vi "SISTEMA INTELIGENTE DE DETECÇÃO DE GAS.vi"() -> ()   [LabVIEW 2020]
uses:
  <vilib>/MakerHub/LINX/Public/Peripherals/Analog/Analog Read 1 Chan.vi
  <vilib>/MakerHub/LINX/Public/Peripherals/Digital/Digital Write 1 Chan.vi
  <vilib>/MakerHub/LINX/Public/Peripherals/Analog/Analog Read N Chans.vi
  <vilib>/MakerHub/LINX/Public/Peripherals/Digital/Digital Write N Chans.vi
  <vilib>/MakerHub/LINX/Private/Local IO/LinxAnalogRead.vi
  <vilib>/MakerHub/LINX/Public/Utilities/Check Channel.vi
  <vilib>/MakerHub/LINX/Private/Local IO/LinxDigitalWrite.vi
  <vilib>/MakerHub/LINX/Public/Utilities/Open Serial.vi
  <vilib>/MakerHub/LINX/Private/Utilties/Generate Error.vi
  <vilib>/MakerHub/LINX/Public/Sensors/Temperature/TMP3x/TMP35.vi
  <vilib>/MakerHub/LINX/LMH-LINX.lvlib
  <vilib>/MakerHub/LINX/Public/Sensors/Temperature/TMP3x/TMP3x.lvlib
panel:
  in  "Tab Control":enum32{"Supervisório", "Configuração"}(tab)
  out "Gráfico da temperatura ambiente":dbl(graph)
  out "2D Picture":picture
  out "Gráfico de gás no ambiente":T1(graph)
  out "ledExp2":bool
  out "ledDep2":bool
  out "ledCoz2":bool
  out "ledCoz1":bool
  out "ledExp1":bool
  out "ledDep1":bool
  out "°C":dbl format="%#_2g"
  out "Cozimento":dbl(knob) scale=0.0..5.0
  out "Expedição":dbl(knob) scale=0.0..5.0
  out "Depósito":dbl(knob) scale=0.0..5.0
  out "Temperatura\nambiente":dbl(slide) scale=0.0..100.0
  out "'ppm'":dbl format="%#_2g"
  out "'ppm'":dbl format="%#_2g"
  out "'ppm'":dbl format="%#_2g"
  in  "fundoAlarme":string
  in  "Set-point gas":fxp<+,64,32>
  in  "Serial Port":refnum<visa-resource-name>="N/A"
  in  "sensorGas1":u8
  in  "sensorGas2":u8
  in  "sensorGas3":u8
  in  "sensorTempLM35":u8
  in  "stop":bool
  in  "saidaSirene":u8
  in  "saidaLuminoso":u8
  in  "diretorioDatalogger":path
  in  "imagemAlertaTemp":path
  in  "Set-point temp":dbl
  in  "imagemNormalidade":path
  in  "imagemAlertaGasTemp":path
  in  "imagemAlertaGas":path
  # "SISTEMA DE MONITORAMENTO DE EMERGÊNCIA"
  # "Planta baixa fábrica alimentícia"
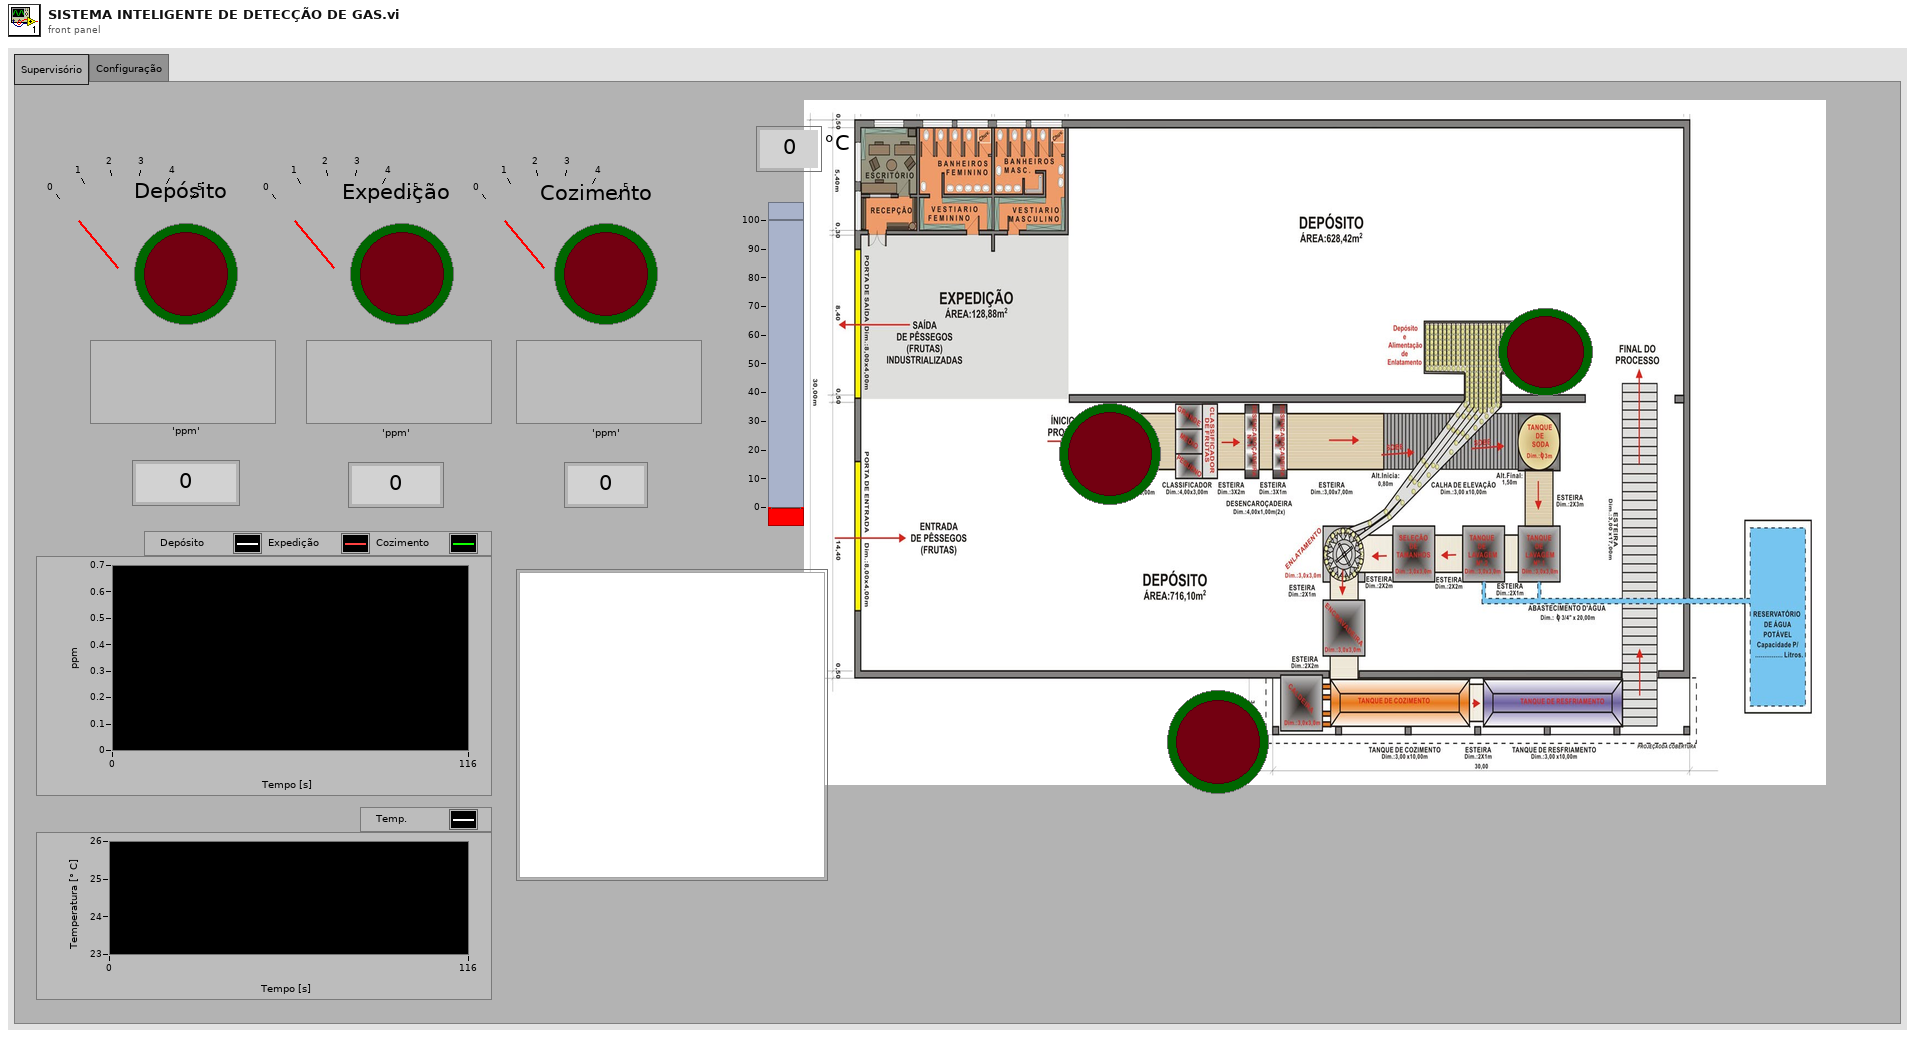
[diagram p1: front panel]
types:
  T1 = cluster{"Depósito":dbl, "Expedição":dbl, "Cozimento":dbl}
  T2 = typedef "LMH-LINX.lvlib/LINX Ref.ctl" = cluster{"IO":T3, "Interface":T4, "LINX Device Config":T5}
  T3 = typedef "LMH-LINX.lvlib/Platform.ctl" = enum16{"Remote", "Local"}
  T4 = typedef "LMH-LINX.lvlib/Interface.ctl" = enum16{"Serial", "TCP"}
  T5 = typedef "LMH-LINX.lvlib/Device.lvlib/LINX Device Config.ctl" = cluster{"Interface":T4, "COM Port":refnum<visa-resource-name>, "TCP Configuration":T6, "Device Family":u8, "Device ID":u8, "Device Name":string, "TCP Ref":refnum<k5>, "Channels":T7}
  T6 = typedef "LMH-LINX.lvlib/Device.lvlib/TCP Config.ctl" = cluster{"IP Address":string, "Port":u16}
  T7 = typedef "LMH-LINX.lvlib/Channels.ctl" = cluster{"DI":u8[], "DO":u8[], "AI":u8[], "AO":u8[], "PWM":u8[], "QE":u8[], "UART":u8[], "I2C 2":u8[], "SPI":u8[], "CAN":u8[], "Servo":u8[], "AI Ref (V)":dbl, "AI Resolution (Bits)":u8, "AO Ref (V)":dbl, "AO Resolution (Bits)":u8}
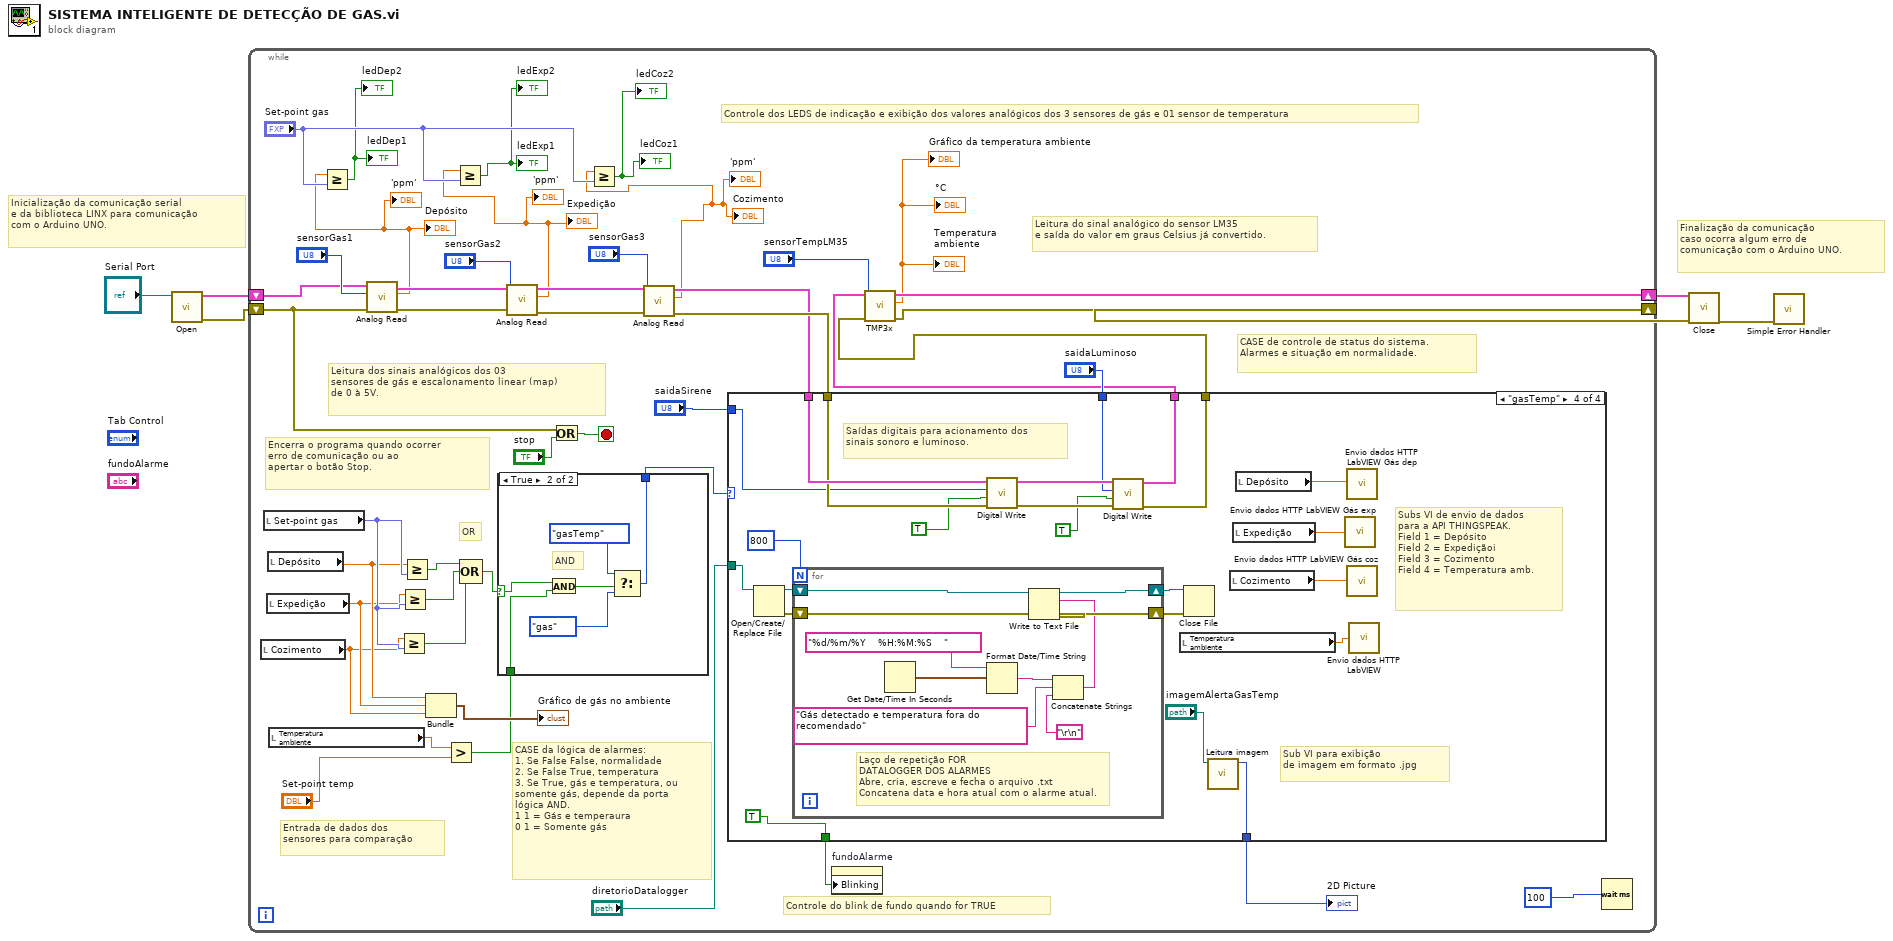
[diagram p0: block diagram]
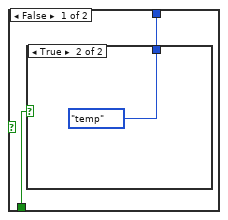
[diagram p2: hidden frame]
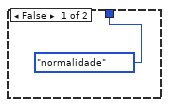
[diagram p3: hidden frame]
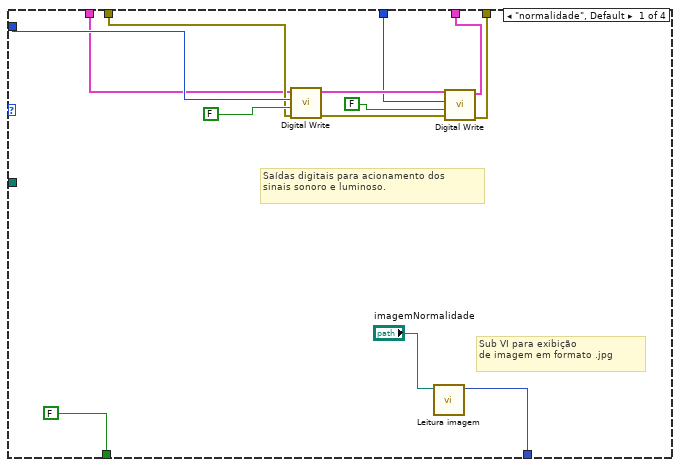
[diagram p4: hidden frame]
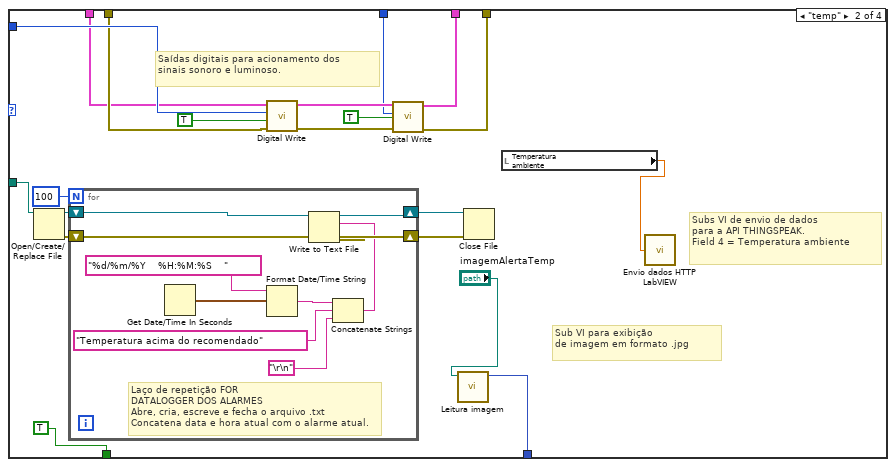
[diagram p5: hidden frame]
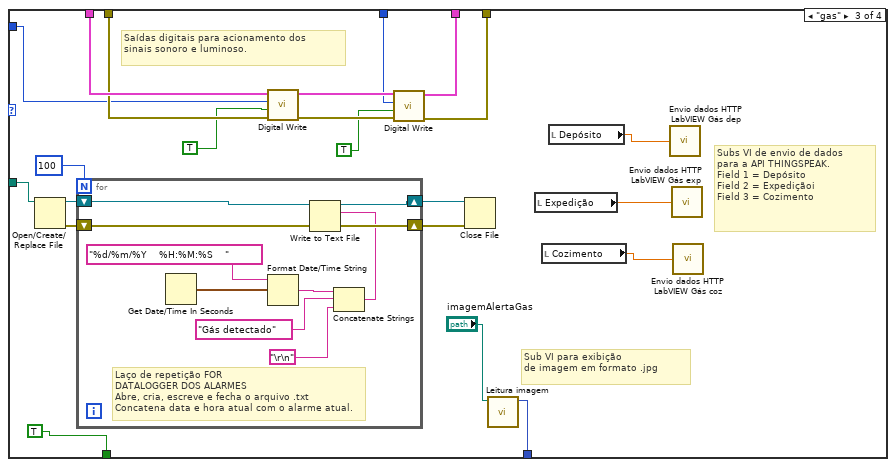
[diagram p6: hidden frame]
diagram:
  # "Finalização da comunicação\ncaso ocorra algum erro de\ncomunicação com o Arduino UNO."
  # "Inicialização da comunicação serial\ne da biblioteca LINX para comunicação \ncom o Arduino UNO."
  n1 = call-poly <vilib>:"Open.vi"("Serial Port"="Serial Port") -> ("Error Out"=w6:errorcluster, "LINX Resource"=w3:T2)  [unwired: 8 in, 1 out]
  n2 = while {
    shift-right: [w50] -> w5
    shift-left: w6 -> [w33]
    shift-right: [w49] -> w2
    shift-left: w3 -> [w34]
    stop <- w48 stop-if-true
    # "Encerra o programa quando ocorrer \nerro de comunicação ou ao \napertar o botão Stop."
    # "Entrada de dados dos\nsensores para comparação"
    # "OR"
    # "CASE de controle de status do sistema. \nAlarmes e situação em normalidade."
    # "Leitura do sinal analógico do sensor LM35 \ne saída do valor em graus Celsius já convertido."
    # "Leitura dos sinais analógicos dos 03\nsensores de gás e escalonamento linear (map)\nde 0 à 5V."
    # "CASE da lógica de alarmes:\n1. Se False False, normalidade\n2. Se False True, temperatura\n3. Se True, gás e temperatura, ou\nsomente gás, depende da porta\nlógica AND.\n1 1 = Gás e temperaura\n0 1 = Somente gás"
    # "Controle do blink de fundo quando for TRUE"
    # "Controle dos LEDS de indicação e exibição dos valores analógicos dos 3 sensores de gás e 01 sensor de temperatura"
    n3 = local read "Cozimento"() -> (w27:dbl)
    n4 = local read "Set-point gas"() -> (w30:fxp<+,64,32>)
    n5 = local read "Expedição"() -> (w28:dbl)
    n6 = local read "Depósito"() -> (w29:dbl)
    n7 = local read "Temperatura\nambiente"() -> (w23:dbl)
    n8 = call-poly <vilib>:"Analog Read.vi"("Error In"=w33, "Analog Channel"="sensorGas1", "LINX Resource"=w34) -> ("Error Out"=w51:errorcluster, "Voltage"=w9:dbl, "LINX Resource"=w45:T2)  [unwired: 5 in, 1 out]
    "Depósito" <- w9
    "'ppm'" <- w9
    n9 = Greater Or Equal?(x=w9, y="Set-point gas") -> (x >= y?=→"ledDep1" →"ledDep2":bool)
    n10 = Greater Or Equal?(x=w27, y=w30) -> (x >= y?=w14:bool)
    n11 = Greater Or Equal?(x=w28, y=w30) -> (x >= y?=w15:bool)
    n12 = Greater Or Equal?(x=w29, y=w30) -> (x >= y?=w16:bool)
    n13 = Bundle("Depósito"=w29, "Expedição"=w28, "Cozimento"=w27) -> (→"Gráfico de gás no ambiente":T1)  [unwired: 1 in]
    n14 = Greater?(x=w23, y="Set-point temp") -> (0:w12:bool)
    n15 = Compound Arithmetic op=OR(w16, w15, w14) -> (w13:bool)
    n16 = case shown="True" w13 {
      selector: w13 -> [_ w59]
      tunnel: [w52 w57] -> w17
      tunnel: w12 -> [w53 w58]
      frame False {
        n17 = case shown="True" w53 {
          tunnel: [enum16{"gasTemp", "normalidade", "temp", "gas"}."normalidade" enum16{"gasTemp", "normalidade", "temp", "gas"}."temp"] -> w52
          frame False {
          }
          frame True {
          }
        }
      }
      frame True {
        # "AND"
        n18 = And(x=w59, y=w58) -> (x .and. y?=w60:bool)
        n19 = Select(t=enum16{"gasTemp", "normalidade", "temp", "gas"}."gasTemp", s=w60, f=enum16{"gasTemp", "normalidade", "temp", "gas"}."gas") -> (s? t:f=w57:enum16{"gasTemp", "normalidade", "temp", "gas"})
      }
    }
    n20 = call-poly <vilib>:"Analog Read.vi"("Error In"=w51, "Analog Channel"="sensorGas2", "LINX Resource"=w45) -> ("Error Out"=w41:errorcluster, "Voltage"=w10:dbl, "LINX Resource"=w40:T2)  [unwired: 5 in, 1 out]
    "Expedição" <- w10
    "'ppm'" <- w10
    n21 = Greater Or Equal?(x=w10, y="Set-point gas") -> (x >= y?=→"ledExp1" →"ledExp2":bool)
    n22 = Or(x=w33, y="stop") -> (x .or. y?=w48:bool)
    n23 = call-poly <vilib>:"Analog Read.vi"("Error In"=w41, "Analog Channel"="sensorGas3", "LINX Resource"=w40) -> ("Error Out"=w22:errorcluster, "Voltage"=w11:dbl, "LINX Resource"=w20:T2)  [unwired: 5 in, 1 out]
    "Cozimento" <- w11
    "'ppm'" <- w11
    n24 = Greater Or Equal?(x=w11, y="Set-point gas") -> (x >= y?=→"ledCoz1" →"ledCoz2":bool)
    n25 = case shown="\"gasTemp\"" w17 {
      tunnel: "saidaSirene" -> [w71 w92 w115 w147]
      tunnel: "saidaLuminoso" -> [w72 w91 w114 w146]
      tunnel: "diretorioDatalogger" -> [_ w90 w116 w149]
      tunnel: w22 -> [w68 w85 w119 w152]
      tunnel: [w65 w84 w117 w151] -> w21
      tunnel: w20 -> [w67 w83 w120 w153]
      tunnel: [w66 w82 w118 w150] -> w19
      tunnel: [FALSE TRUE TRUE TRUE] -> w18
      tunnel: [w63 w75 w106 w138] -> w8
      frame "normalidade", Default {
        # "Sub VI para exibição\nde imagem em formato .jpg"
        # "Saídas digitais para acionamento dos\nsinais sonoro e luminoso."
        n26 = call-poly <vilib>:"Digital Write.vi"("Error In"=w68, "Output Value"=FALSE, "DO Channel"=w71, "LINX Resource"=w67) -> ("Error Out"=w73:errorcluster, "LINX Resource"=w74:T2)  [unwired: 6 in]
        n27 = call "Leitura imagem.vi"("path to JPEG file"="imagemNormalidade") -> ("new picture"=w63:picture)  [unwired: 10 in]
        n28 = call-poly <vilib>:"Digital Write.vi"("Error In"=w73, "Output Value"=FALSE, "DO Channel"=w72, "LINX Resource"=w74) -> ("Error Out"=w65:errorcluster, "LINX Resource"=w66:T2)  [unwired: 6 in]
      }
      frame "temp" {
        # "Sub VI para exibição\nde imagem em formato .jpg"
        # "Saídas digitais para acionamento dos\nsinais sonoro e luminoso."
        # "Subs VI de envio de dados\npara a API THINGSPEAK.\nField 4 = Temperatura ambiente"
        n29 = Open/Create/Replace File(file path (use dialog)=w90) -> (refnum out=w89:refnum<file>, error out=w86:errorcluster)  [unwired: 5 in, 1 out]
        n30 = for {
          N: 100 -> [_]
          shift-right: [w103] -> w88
          shift-left: w89 -> [w104]
          shift-right: [w102] -> w87
          shift-left: w86 -> [w101]
          # "Laço de repetição FOR\nDATALOGGER DOS ALARMES\nAbre, cria, escreve e fecha o arquivo .txt\nConcatena data e hora atual com o alarme atual."
          n31 = Get Date/Time In Seconds() -> (seconds since 1Jan1904=w100:timestamp)
          n32 = Format Date/Time String(time format string (%c)="%d/%m/%Y    %H:%M:%S    ", seconds (now)=w100) -> (date/time string=w98:string)  [unwired: 1 in]
          n33 = Concatenate Strings(w98, "Temperatura acima do recomendado", "\r\n") -> (w97:string)
          n34 = Write to Text File(file (use dialog)=w104, text=w97, error in=w101) -> (refnum out=w103:refnum<file>, error out=w102:errorcluster)  [unwired: 1 in, 1 out]
        }
        n35 = call-poly <vilib>:"Digital Write.vi"("Error In"=w85, "Output Value"=TRUE, "DO Channel"=w92, "LINX Resource"=w83) -> ("Error Out"=w94:errorcluster, "LINX Resource"=w93:T2)  [unwired: 6 in]
        n36 = call-poly <vilib>:"Digital Write.vi"("Error In"=w94, "Output Value"=TRUE, "DO Channel"=w91, "LINX Resource"=w93) -> ("Error Out"=w84:errorcluster, "LINX Resource"=w82:T2)  [unwired: 6 in]
        n37 = call "Leitura imagem.vi"("path to JPEG file"="imagemAlertaTemp") -> ("new picture"=w75:picture)  [unwired: 10 in]
        n38 = Close File(refnum=w88, error in=w87) -> ()  [unwired: 2 out]
        n39 = local read "Temperatura\nambiente"() -> (w77:dbl)
        n40 = call "Envio dados HTTP LabVIEW.vi"("valorAnalogicoTemp"=w77) -> ()  [unwired: 1 in]
      }
      frame "gas" {
        # "Sub VI para exibição\nde imagem em formato .jpg"
        # "Saídas digitais para acionamento dos\nsinais sonoro e luminoso."
        # "Subs VI de envio de dados\npara a API THINGSPEAK.\nField 1 = Depósito\nField 2 = Expediçãoi\nField 3 = Cozimento"
        n41 = Open/Create/Replace File(file path (use dialog)=w116) -> (refnum out=w123:refnum<file>, error out=w126:errorcluster)  [unwired: 5 in, 1 out]
        n42 = for {
          N: 100 -> [_]
          shift-right: [w135] -> w125
          shift-left: w126 -> [w136]
          shift-right: [w134] -> w124
          shift-left: w123 -> [w133]
          # "Laço de repetição FOR\nDATALOGGER DOS ALARMES\nAbre, cria, escreve e fecha o arquivo .txt\nConcatena data e hora atual com o alarme atual."
          n43 = Get Date/Time In Seconds() -> (seconds since 1Jan1904=w132:timestamp)
          n44 = Format Date/Time String(time format string (%c)="%d/%m/%Y    %H:%M:%S    ", seconds (now)=w132) -> (date/time string=w130:string)  [unwired: 1 in]
          n45 = Concatenate Strings(w130, "Gás detectado", "\r\n") -> (w129:string)
          n46 = Write to Text File(file (use dialog)=w133, text=w129, error in=w136) -> (refnum out=w134:refnum<file>, error out=w135:errorcluster)  [unwired: 1 in, 1 out]
        }
        n47 = call-poly <vilib>:"Digital Write.vi"("Error In"=w119, "Output Value"=TRUE, "DO Channel"=w115, "LINX Resource"=w120) -> ("Error Out"=w121:errorcluster, "LINX Resource"=w122:T2)  [unwired: 6 in]
        n48 = call-poly <vilib>:"Digital Write.vi"("Error In"=w121, "Output Value"=TRUE, "DO Channel"=w114, "LINX Resource"=w122) -> ("Error Out"=w117:errorcluster, "LINX Resource"=w118:T2)  [unwired: 6 in]
        n49 = Close File(refnum=w124, error in=w125) -> ()  [unwired: 2 out]
        n50 = call "Leitura imagem.vi"("path to JPEG file"="imagemAlertaGas") -> ("new picture"=w106:picture)  [unwired: 10 in]
        n51 = local read "Expedição"() -> (w108:dbl)
        n52 = local read "Cozimento"() -> (w107:dbl)
        n53 = local read "Depósito"() -> (w109:dbl)
        n54 = call "Envio dados HTTP LabVIEW Gás dep.vi"("valorAnalogicoTemp"=w109) -> ()  [unwired: 1 in]
        n55 = call "Envio dados HTTP LabVIEW Gás exp.vi"("valorAnalogicoTemp"=w108) -> ()  [unwired: 1 in]
        n56 = call "Envio dados HTTP LabVIEW Gás coz.vi"("valorAnalogicoTemp"=w107) -> ()  [unwired: 1 in]
      }
      frame "gasTemp" {
        # "Sub VI para exibição\nde imagem em formato .jpg"
        # "Saídas digitais para acionamento dos\nsinais sonoro e luminoso."
        # "Subs VI de envio de dados\npara a API THINGSPEAK.\nField 1 = Depósito\nField 2 = Expediçãoi\nField 3 = Cozimento\nField 4 = Temperatura amb."
        n57 = Open/Create/Replace File(file path (use dialog)=w149) -> (refnum out=w156:refnum<file>, error out=w159:errorcluster)  [unwired: 5 in, 1 out]
        n58 = for {
          N: 800 -> [_]
          shift-right: [w168] -> w158
          shift-left: w159 -> [w169]
          shift-right: [w167] -> w157
          shift-left: w156 -> [w166]
          # "Laço de repetição FOR\nDATALOGGER DOS ALARMES\nAbre, cria, escreve e fecha o arquivo .txt\nConcatena data e hora atual com o alarme atual."
          n59 = Get Date/Time In Seconds() -> (seconds since 1Jan1904=w165:timestamp)
          n60 = Format Date/Time String(time format string (%c)="%d/%m/%Y    %H:%M:%S    ", seconds (now)=w165) -> (date/time string=w163:string)  [unwired: 1 in]
          n61 = Concatenate Strings(w163, "Gás detectado e temperatura fora do recomendado", "\r\n") -> (w162:string)
          n62 = Write to Text File(file (use dialog)=w166, text=w162, error in=w169) -> (refnum out=w167:refnum<file>, error out=w168:errorcluster)  [unwired: 1 in, 1 out]
        }
        n63 = call-poly <vilib>:"Digital Write.vi"("Error In"=w152, "Output Value"=TRUE, "DO Channel"=w147, "LINX Resource"=w153) -> ("Error Out"=w154:errorcluster, "LINX Resource"=w155:T2)  [unwired: 6 in]
        n64 = call-poly <vilib>:"Digital Write.vi"("Error In"=w154, "Output Value"=TRUE, "DO Channel"=w146, "LINX Resource"=w155) -> ("Error Out"=w151:errorcluster, "LINX Resource"=w150:T2)  [unwired: 6 in]
        n65 = local read "Temperatura\nambiente"() -> (w140:dbl)
        n66 = Close File(refnum=w157, error in=w158) -> ()  [unwired: 2 out]
        n67 = call "Leitura imagem.vi"("path to JPEG file"="imagemAlertaGasTemp") -> ("new picture"=w138:picture)  [unwired: 10 in]
        n68 = local read "Cozimento"() -> (w141:dbl)
        n69 = local read "Expedição"() -> (w139:dbl)
        n70 = local read "Depósito"() -> (w142:dbl)
        n71 = call "Envio dados HTTP LabVIEW Gás exp.vi"("valorAnalogicoTemp"=w139) -> ()  [unwired: 1 in]
        n72 = call "Envio dados HTTP LabVIEW Gás dep.vi"("valorAnalogicoTemp"=w142) -> ()  [unwired: 1 in]
        n73 = call "Envio dados HTTP LabVIEW Gás coz.vi"("valorAnalogicoTemp"=w141) -> ()  [unwired: 1 in]
        n74 = call "Envio dados HTTP LabVIEW.vi"("valorAnalogicoTemp"=w140) -> ()  [unwired: 1 in]
      }
    }
    "2D Picture" <- w8
    n75 = property on="fundoAlarme" class="Str"("Blinking"=w18) -> ()  [unwired: 2 in, 2 out]
    n76 = call-poly <vilib>:"TMP3x.vi"("Error In"=w21, "Analog Channel"="sensorTempLM35", "LINX Resource"=w19) -> ("Error Out"=w50:errorcluster, "Temp C"=→"Temperatura\nambiente" →"°C" →"Gráfico da temperatura ambiente":dbl, "LINX Resource"=w49:T2)  [unwired: 6 in]
    n77 = Wait (ms)(milliseconds to wait=u32 100) -> ()  [unwired: 1 out]
  }
  n78 = call <vilib>:"Close.vi"("Error In"=w5, "LINX Resource"=w2) -> ("Error Out"=w1:errorcluster)  [unwired: 9 in]
  n79 = call <vilib>:"Simple Error Handler.vi"("error in (no error)"=w1) -> ()  [unwired: 4 in, 5 out]
